vi "read keys per section.vi"(7 "section":string, 8 "error in (no error)":errorcluster, 11 "Refnum in":T2) -> (0 "error out":errorcluster, 2 "section data":T1, 3 "Refnum out":T2)   [LabVIEW 2024, in "API Path Config Files Management.lvlib"]
doc: "This function retrieves all keys and their corresponding values from a specified section in a configuration .ini file. The output is a cluster containing three elements: a string for the section name, a 1-D string array for the keys, and a 1-D string array for the corresponding values."
uses:
  API Path Config Files Management.lvlib
  <vilib>/Utility/config.llb/Config Data RefNum.ctl
  section data path.ctl
  <vilib>/Utility/config.llb/Read Key (String).vi
  <vilib>/Utility/config.llb/NI_LVConfig.lvlib
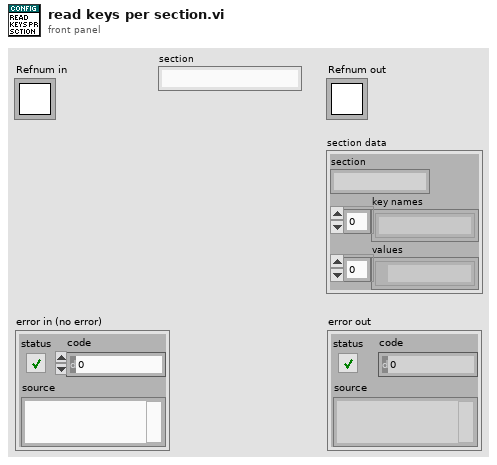
[diagram p1: front panel]
types:
  T1 = typedef "API Path Config Files Management.lvlib/section data path.ctl" = cluster{"section":string, "key names":string[], "values":path[]}
  T2 = typedef "NI_LVConfig.lvlib/Config Data RefNum.ctl" = refnum<k1>
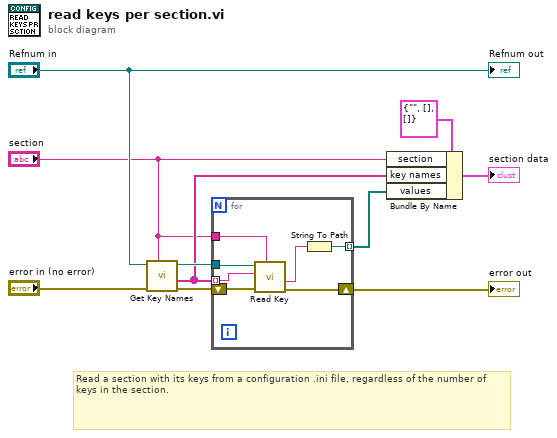
[diagram p0: block diagram]
diagram:
  # "Read a section with its keys from a configuration .ini file, regardless of the number of keys in the section."
  n1 = call <vilib>:"Get Key Names.vi"("section"="section", "error in (no error)"="error in (no error)", "refnum"="Refnum in") -> ("error out"=w8:errorcluster, "key names"=w3:string[], "refnum out"=w7:T2)  [unwired: 5 in, 1 out]
  n2 = for {
    tunnel: w3 -> [w16] mode=indexing
    tunnel: w7 -> [w17]
    tunnel: "section" -> [w15]
    tunnel: [w11] -> w4 mode=indexing
    shift-right: [w12] -> w9
    shift-left: w8 -> [w13]
    n3 = call-poly <vilib>:"Read Key.vi"("section"=w15, "error in (no error)"=w13, "key"=w16, "refnum"=w17) -> ("error out"=w12:errorcluster, "value"=w14:string)  [unwired: 4 in, 2 out]
    n4 = String To Path(string=w14) -> (path=w11:path)
  }
  "error out" <- w9
  n5 = Bundle By Name(cluster=T1 {"section"="", "key names"=[], "values"=[]} ("section data"), "section"="section", "key names"=w3, "values"=w4) -> (→"section data":T1)
  "Refnum out" <- "Refnum in"
